vi "FABR-Options Dialog.vi"(0 "Params In":T2={"Stimulus"={"Destination"="", "Rep rate (/sec)"=30.0, "Alternate Polarity"=FALSE, "Duration (ms)"=0.0, "Ramp (ms)"=16.0, "Fs (Hz)"=5.0, "Frame size (s)"=0.0}, "Sequence"={"Freq"={"Start (kHz)"=20.0, "Stop (kHz)"=80.0, "Step (oct)"=5.0, "Skip (oct)"=0.0}, "Level"={"Start (dB)"=20, "Stop (dB)"=80, "Step (dB)"=5}, "Order"=enum."Interleaved"}, "Response"={"Gain"=10000.0, "Averages"=512, "Window (ms)"=8.5, "Fs (Hz)"=25000.0, "Save raw"=FALSE}, "Reject"=0.0} {"Sequence"."Level"."Start (dB)" step=5; "Sequence"."Freq"."Start (kHz)" step=5.0; "Response"."Window (ms)" format="%.2f"}, 2 "Parent VI":refnum<vi>, 5 "Threshold Estimation In":T7) -> (4 "Params Out":T2={"Stimulus"={"Destination"="", "Rep rate (/sec)"=30.0, "Alternate Polarity"=FALSE, "Duration (ms)"=0.0, "Ramp (ms)"=16.0, "Fs (Hz)"=5.0, "Frame size (s)"=0.0}, "Sequence"={"Freq"={"Start (kHz)"=20.0, "Stop (kHz)"=80.0, "Step (oct)"=5.0, "Skip (oct)"=0.0}, "Level"={"Start (dB)"=20, "Stop (dB)"=80, "Step (dB)"=5}, "Order"=enum."Interleaved"}, "Response"={"Gain"=10000.0, "Averages"=512, "Window (ms)"=8.5, "Fs (Hz)"=25000.0, "Save raw"=FALSE}, "Reject"=0.0} {"Sequence"."Level"."Start (dB)" step=5; "Sequence"."Freq"."Start (kHz)" step=5.0; "Response"."Window (ms)" format="%.2f"}, 6 "Threshold Estimation Out":T7, 8 "Canceled?":bool)   [LabVIEW 2020]
uses:
  Threshold Estimation VIs/ABR3-Threshold Estimation Parameters.ctl
  Typedefs/FABR-Parameters.ctl
  Typedefs/FABR-Stimulus.ctl
  Typedefs/FABR-Sequence.ctl
  Typedefs/FABR-Order.ctl
  Typedefs/FABR-Response.ctl
  epl-vi-lib/Utility VIs/Buttons/KCheckmarkBoolean 2.ctl
panel:
  in  "Save raw":T1
  in  "Frame size":dbl caption="Frame size (s)"
  in  "AI Fs":dbl caption="Input sampling rate (Hz)"
  in  "R2 criterion":dbl caption="Adj R2 criterion"
  in  "CC criterion":dbl caption="Corrcoef criterion"
  in  "Thr Tmax":dbl caption="Tmax (ms)"
  in  "Thr Tmin":dbl caption="Tmin (ms)"
  in  "ToneRamp":dbl caption="Tone burst ramp length (ms)"
  in  "ToneDur":dbl caption="Tone burst duration (ms)"
  in  "AO Fs":dbl caption="Output sampling rate (Hz)"
  in  "Cancel":bool
  in  "OK":bool
  # "Threshold estimation"
  # "Warning! Unless you're sure you know what you're doing, don't change these parameters"
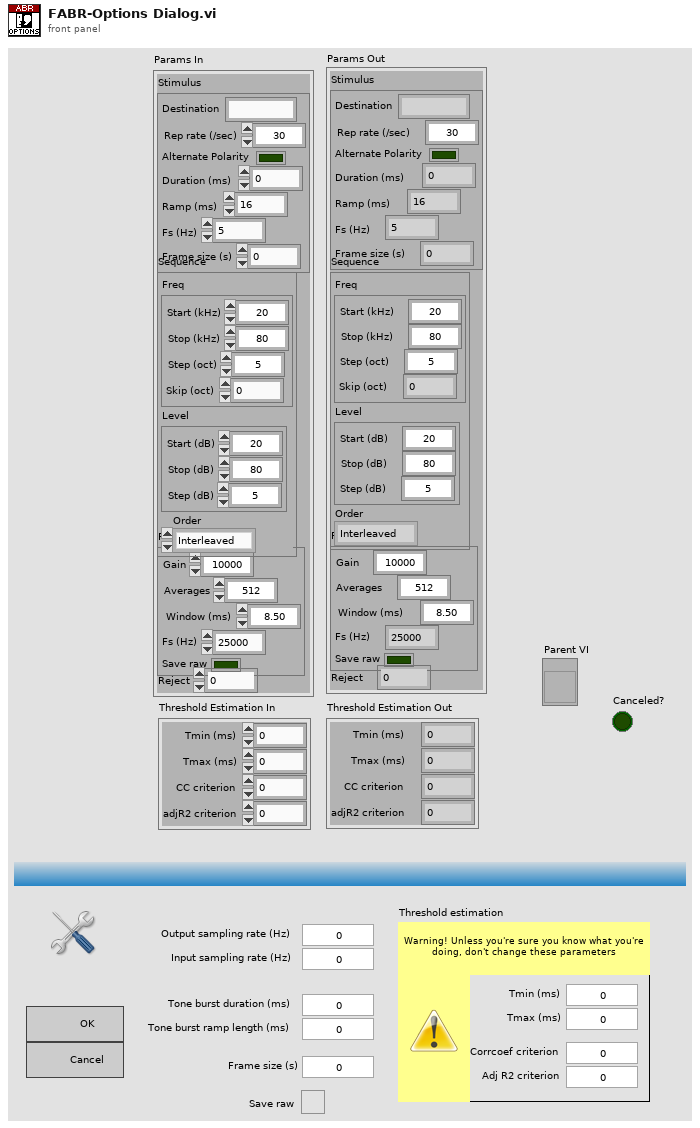
[diagram p1: front panel]
types:
  T1 = typedef "KCheckmarkBoolean 2.ctl" = bool
  T2 = typedef "FABR-Parameters.ctl" = cluster{"Stimulus":T3, "Sequence":T4, "Response":T6, "Reject":dbl}
  T3 = typedef "FABR-Stimulus.ctl" = cluster{"Destination":string, "Rep rate (/sec)":dbl, "Alternate Polarity":bool, "Duration (ms)":dbl, "Ramp (ms)":dbl, "Fs (Hz)":dbl, "Frame size (s)":dbl}
  T4 = typedef "FABR-Sequence.ctl" = cluster{"Freq":cluster{"Start (kHz)":dbl, "Stop (kHz)":dbl, "Step (oct)":dbl, "Skip (oct)":dbl}, "Level":cluster{"Start (dB)":i32, "Stop (dB)":i32, "Step (dB)":i32}, "Order":T5}
  T5 = typedef "FABR-Order.ctl" = enum16{"Interleaved"}
  T6 = typedef "FABR-Response.ctl" = cluster{"Gain":dbl, "Averages":i32, "Window (ms)":sgl, "Fs (Hz)":dbl, "Save raw":bool}
  T7 = typedef "ABR3-Threshold Estimation Parameters.ctl" = cluster{"Tmin (ms)":dbl, "Tmax (ms)":dbl, "CC criterion":dbl, "adjR2 criterion":dbl}
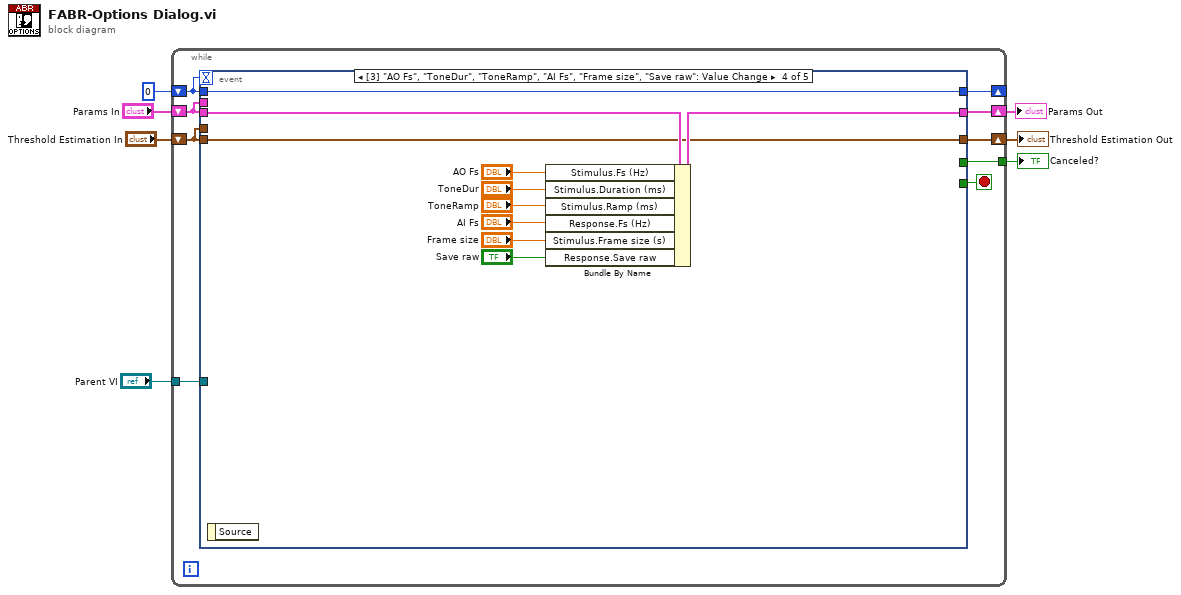
[diagram p0: block diagram]
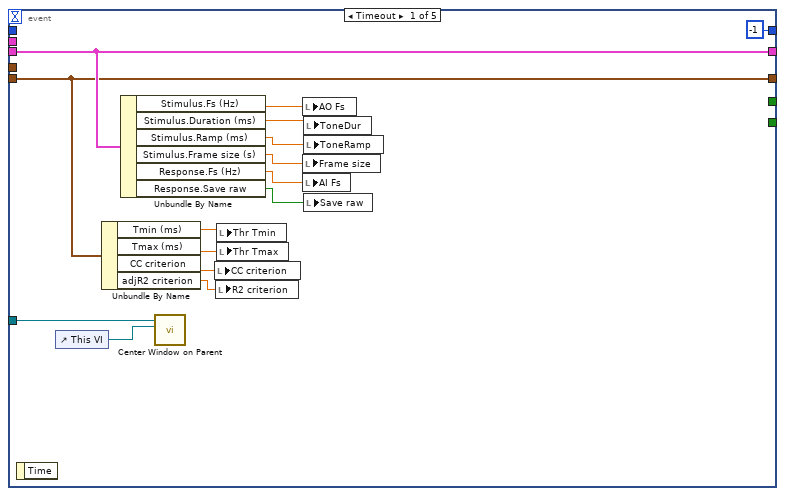
[diagram p2: hidden frame]
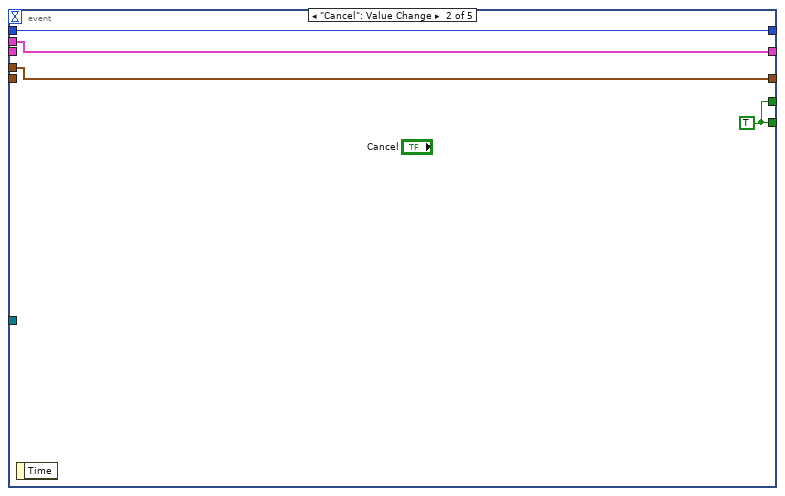
[diagram p3: hidden frame]
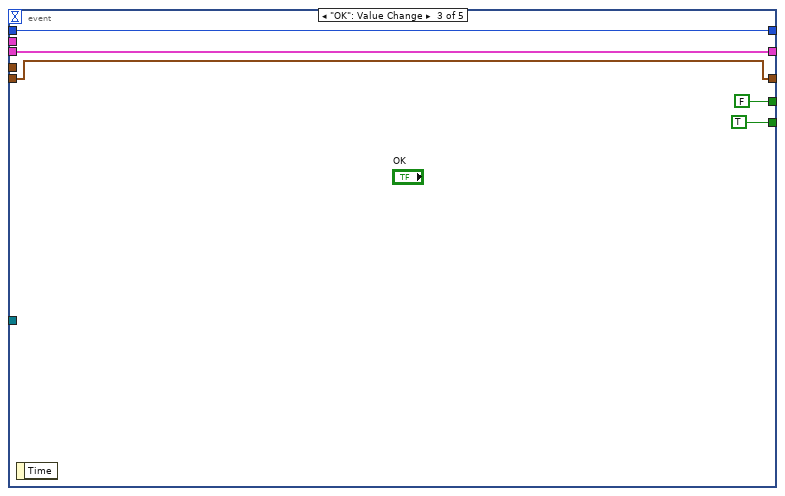
[diagram p4: hidden frame]
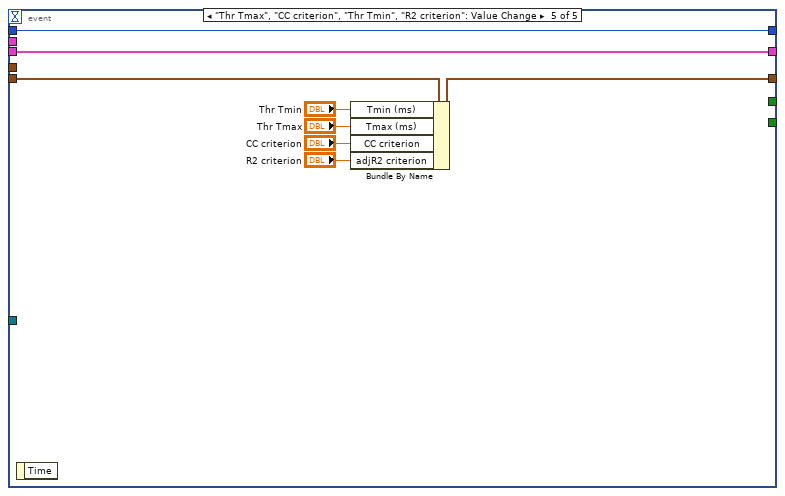
[diagram p5: hidden frame]
diagram:
  n1 = while {
    shift-right: [w16] -> _
    shift-left: 0 -> [w9]
    tunnel: [w13] -> w6
    shift-right: [w15] -> w1
    shift-left: "Params In" -> [w12]
    shift-right: [w11] -> w4
    shift-left: "Threshold Estimation In" -> [w10]
    tunnel: "Parent VI" -> [w8]
    stop <- w14 stop-if-true
    n2 = event shown="[3] \"AO Fs\", \"ToneDur\", \"ToneRamp\", \"AI Fs\", \"Frame size\", \"Save raw\": Value Change" {
      selector: _ -> [_ _ _ _ _]
      dyn-events: _ -> [_ _ _ _ _]
      timeout: w9 -> [_ _ _ _ _]
      tunnel: [-1 w32 w36 w44 w54] -> w16
      tunnel: w12 -> [w30 _ w40 w50 w58]
      tunnel: [w30 w34 w40 w49 w58] -> w15
      tunnel: [_ w35 TRUE _ _] -> w14
      tunnel: [_ w35 FALSE _ _] -> w13
      tunnel: w12 -> [_ w34 _ _ _]
      tunnel: w10 -> [w26 _ w37 w45 w52]
      tunnel: [w26 w33 w37 w45 w51] -> w11
      tunnel: w10 -> [_ w33 _ _ _]
      tunnel: w9 -> [_ w32 w36 w44 w54]
      tunnel: w8 -> [w22 _ _ _ _]
      event Timeout {
        n3 = event-data() -> ()  [unwired: 1 in, 1 out]
        n4 = control-ref of="This VI"() -> (w21:refnum<vi>)
        n5 = Unbundle By Name(w26) -> ("Tmin (ms)"=w25:dbl, "Tmax (ms)"=w24:dbl, "CC criterion"=w23:dbl, "adjR2 criterion"=w20:dbl)
        n6 = Unbundle By Name(w30) -> ("Stimulus.Fs (Hz)"=w29:dbl, "Stimulus.Duration (ms)"=w28:dbl, "Stimulus.Ramp (ms)"=w27:dbl, "Stimulus.Frame size (s)"=w18:dbl, "Response.Fs (Hz)"=w19:dbl, "Response.Save raw"=w17:bool)
        n7 = call "Center Window on Parent.vi"("Parent VI"=w21, "VI in"=w22) -> ()  [unwired: 8 in, 2 out]
        n8 = local write "CC criterion"(w23) -> ()
        n9 = local write "R2 criterion"(w20) -> ()
        n10 = local write "Thr Tmin"(w25) -> ()
        n11 = local write "Thr Tmax"(w24) -> ()
        n12 = local write "AO Fs"(w29) -> ()
        n13 = local write "Frame size"(w18) -> ()
        n14 = local write "AI Fs"(w19) -> ()
        n15 = local write "ToneDur"(w28) -> ()
        n16 = local write "ToneRamp"(w27) -> ()
        n17 = local write "Save raw"(w17) -> ()
      }
      event "Cancel": Value Change {
        w35 = TRUE
        n18 = event-data() -> ()  [unwired: 1 in, 1 out]
      }
      event "OK": Value Change {
        n19 = event-data() -> ()  [unwired: 1 in, 1 out]
      }
      event "AO Fs", "ToneDur", "ToneRamp", "AI Fs", "Frame size": Value Change {
        n20 = event-data() -> ()  [unwired: 1 in, 1 out]
        n21 = Bundle By Name(cluster=w50, "Stimulus.Fs (Hz)"="AO Fs", "Stimulus.Duration (ms)"="ToneDur", "Stimulus.Ramp (ms)"="ToneRamp", "Response.Fs (Hz)"="AI Fs", "Stimulus.Frame size (s)"="Frame size", "Response.Save raw"="Save raw") -> (w49:T2)
      }
      event "Thr Tmax", "CC criterion", "Thr Tmin", "R2 criterion": Value Change {
        n22 = event-data() -> ()  [unwired: 1 in, 1 out]
        n23 = Bundle By Name(cluster=w52, "Tmin (ms)"="Thr Tmin", "Tmax (ms)"="Thr Tmax", "CC criterion"="CC criterion", "adjR2 criterion"="R2 criterion") -> (w51:T7)
      }
    }
  }
  "Canceled?" <- w6
  "Threshold Estimation Out" <- w4
  "Params Out" <- w1
